vi "Init_graphe.vi"() -> ()   [LabVIEW 2015]
uses:
  <vilib>/Utility/miscctls.llb/LVRowAndColumnTypeDef.ctl
  <vilib>/Utility/file.llb/Read From Spreadsheet File (string).vi
panel:
  in  "Horodatage":timestamp
  in  "Bouton Aide":bool
  in  "Quit":bool
  out "horodatage_ok":timestamp
  in  "Fichier données":path
  out "Colonne données brutes":string="0"
  out "Ligne données brutes":string="0"
  out "Noms variables":string[](array[string])
  out "Séparateur fichier brute":string
  in  "Valider":bool
  in  "Nouveau format date":bool
  in  "Format d'horodatage":string(combo)="\"%Y-%m-%d %H:%M:%S\""
  in  "Convertir Horodatage":bool
  out "Nb lignes":i32
  in  "Séparateur":u16(ring)=1 items=["", ",", ";", ".", "Tab", "Espace", ":"]
  out "Horodatage_1":timestamp[](array[timestamp]) format="%<%X\n%x>T"
  out "Table":string[][](table)
  out "Donnees":dbl[][](array[numeric])
  in  "Bouton vide 2":bool
  # "Facultatif : \nSélectionner la dernière cellule des noms de variables  en appuyant sur la touche CTRL"
  # "Sélectionner la 1ère cellule\ndes noms de variables"
  # "Sélectionner la 1ère cellule\nd'horodatage"
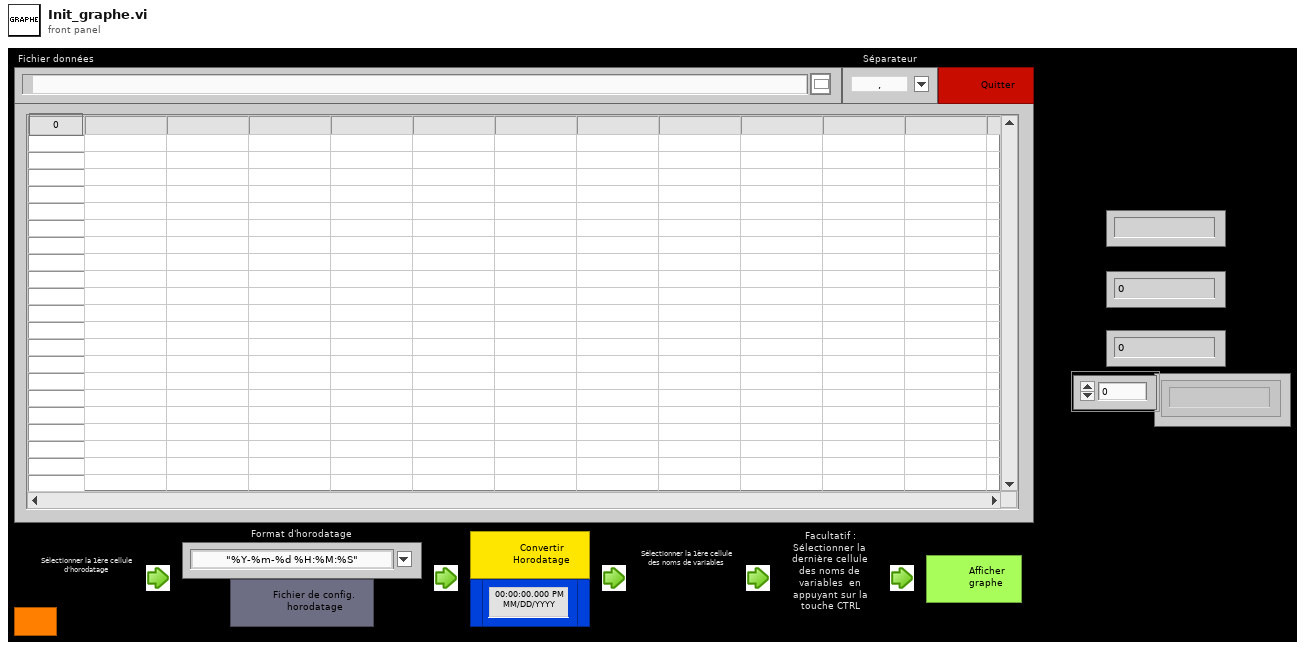
[diagram p1: front panel]
types:
  T1 = typedef "LVRowAndColumnTypeDef.ctl" = cluster{"Row":i32, "Column":i32}
  T2 = typedef "excel Object Reference.ctl" = refnum<k1>
  T3 = enum16{"Left Button", "Center Button", "Right Button", "Window Close"}
  T4 = cluster{"Shift":bool, "Ctrl":bool, "Alt":bool, "Cmd":bool, "Opt":bool}
  T5 = cluster{"Horodatage":timestamp[], "Donnees":dbl[]}[]
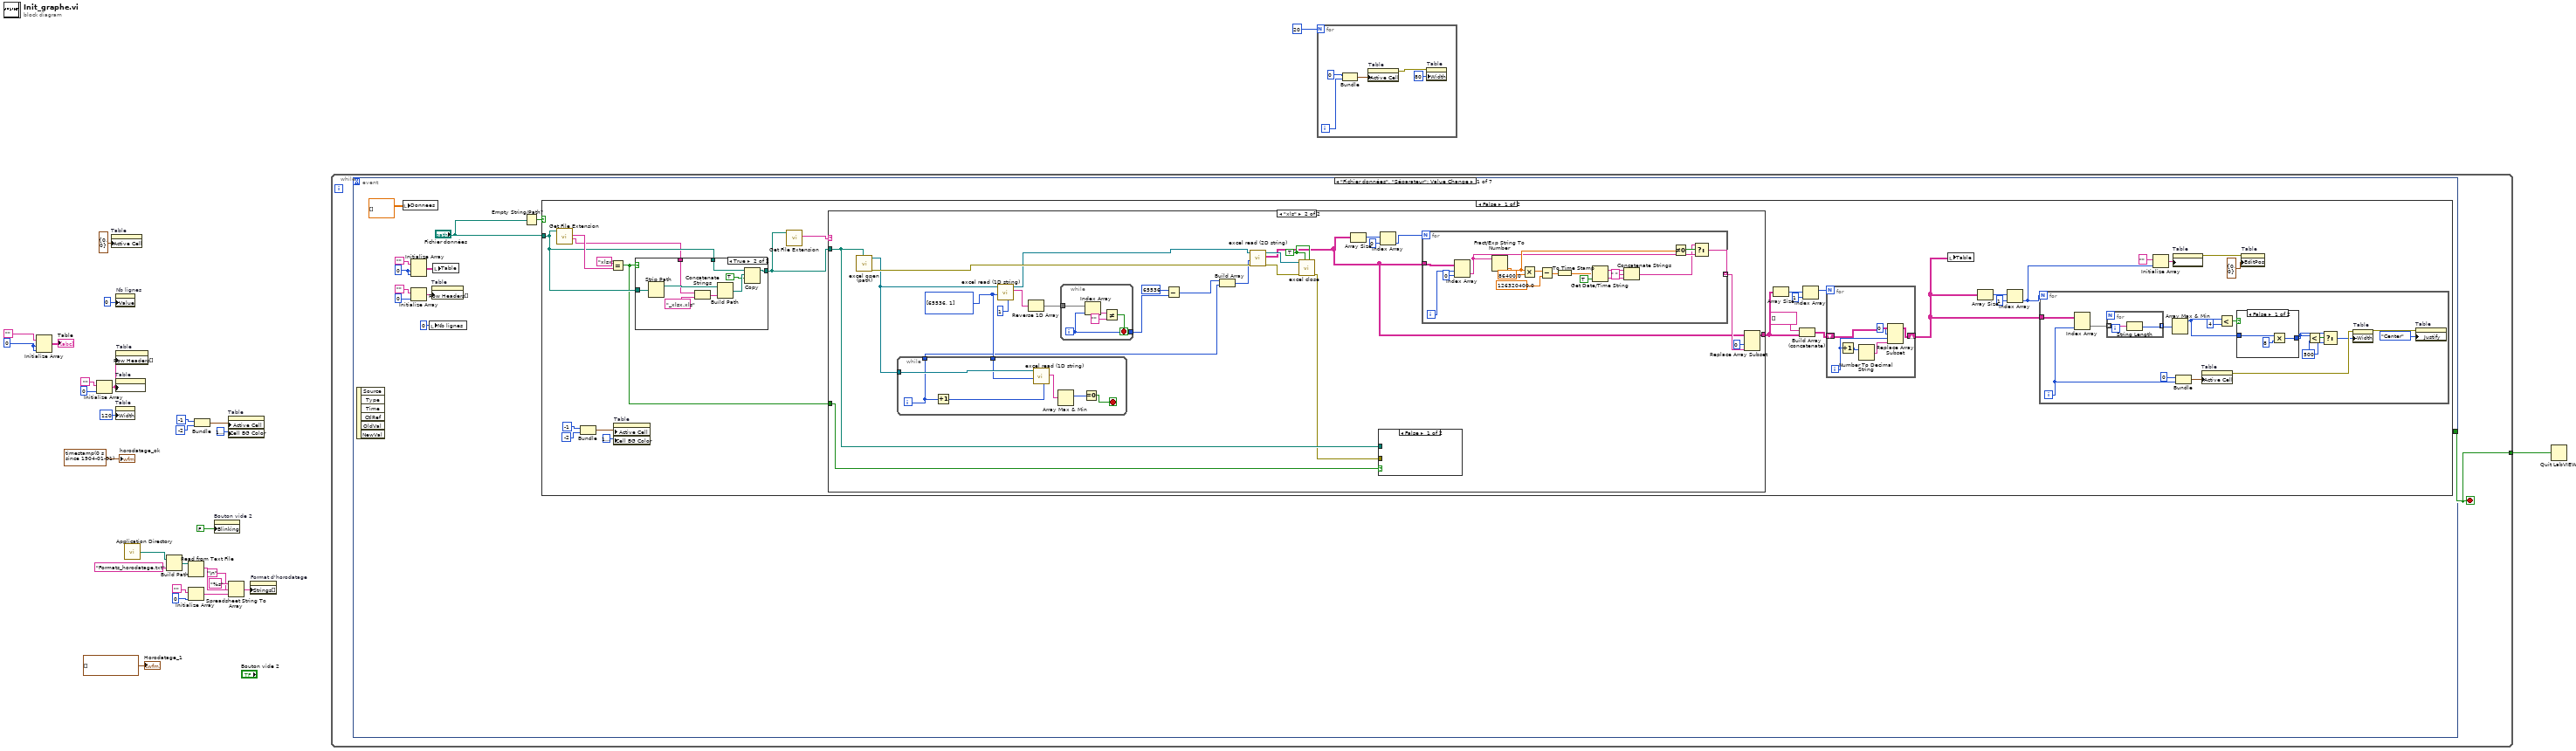
[diagram p0: block diagram]
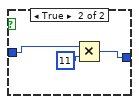
[diagram p3: hidden frame]
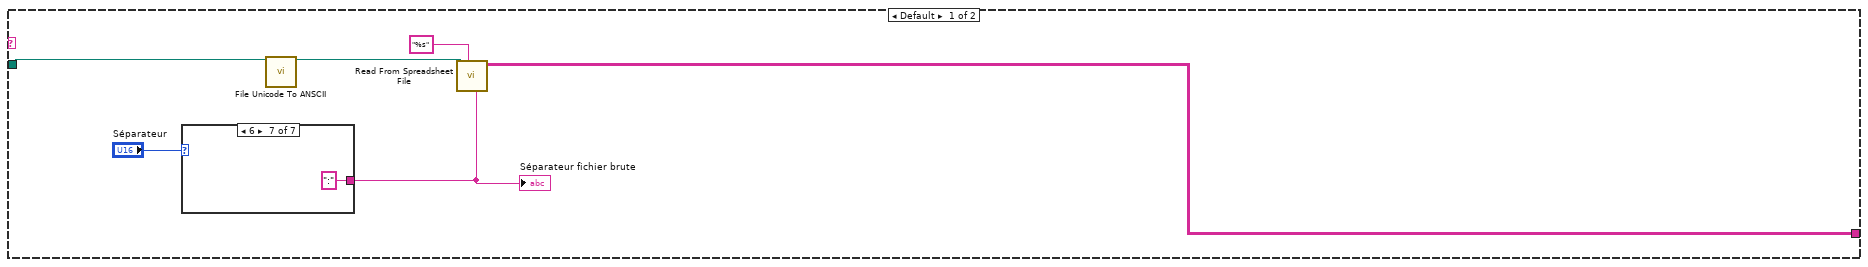
[diagram p4: hidden frame]
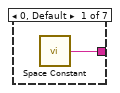
[diagram p5: hidden frame]
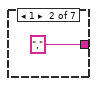
[diagram p6: hidden frame]
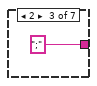
[diagram p7: hidden frame]
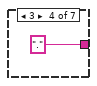
[diagram p8: hidden frame]
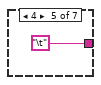
[diagram p9: hidden frame]
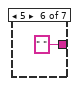
[diagram p10: hidden frame]
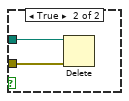
[diagram p11: hidden frame]
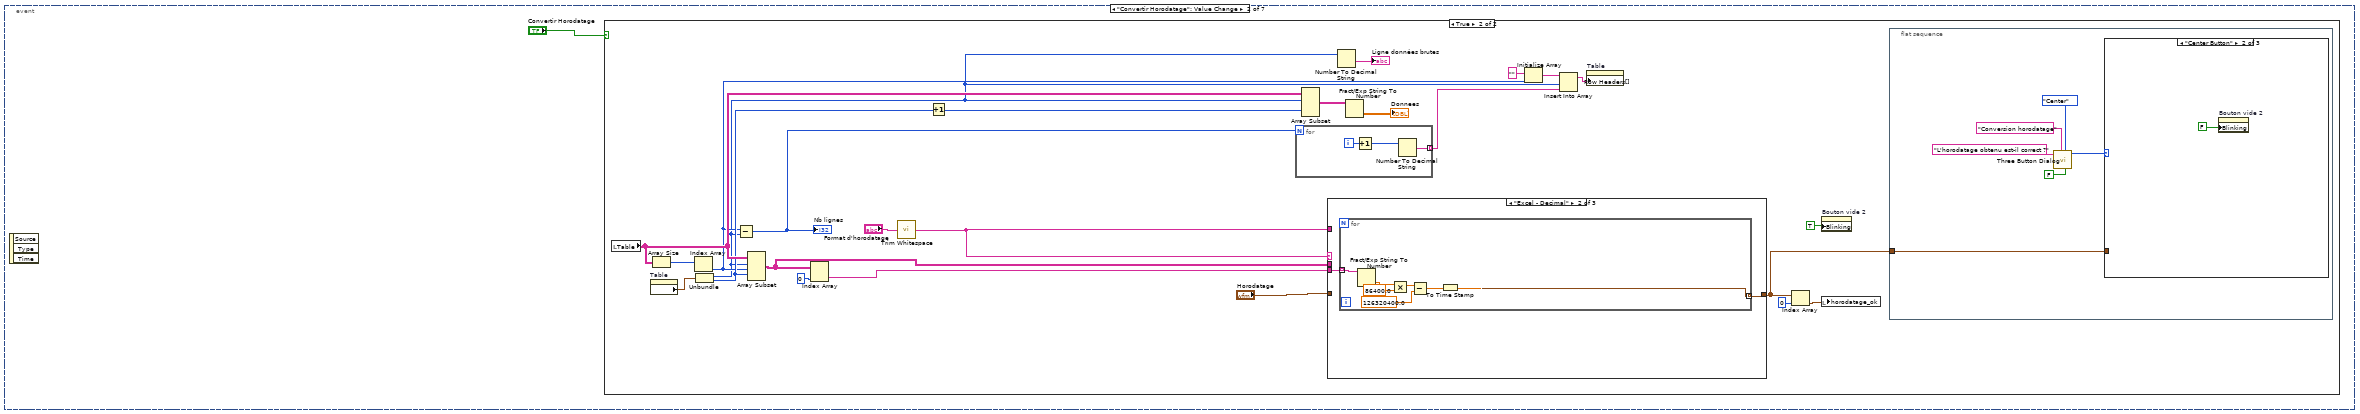
[diagram p13: hidden frame]
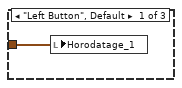
[diagram p15: hidden frame]
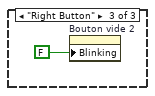
[diagram p16: hidden frame]
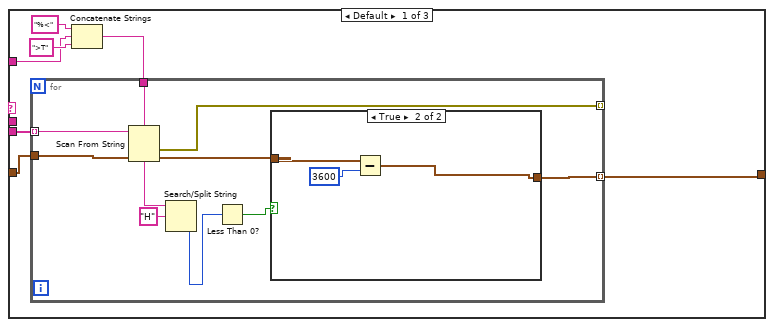
[diagram p17: hidden frame]
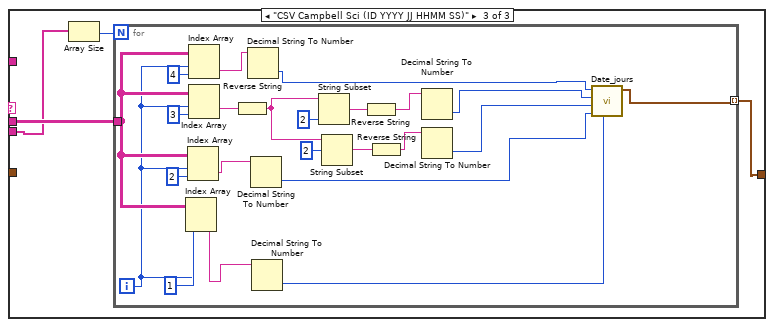
[diagram p19: hidden frame]
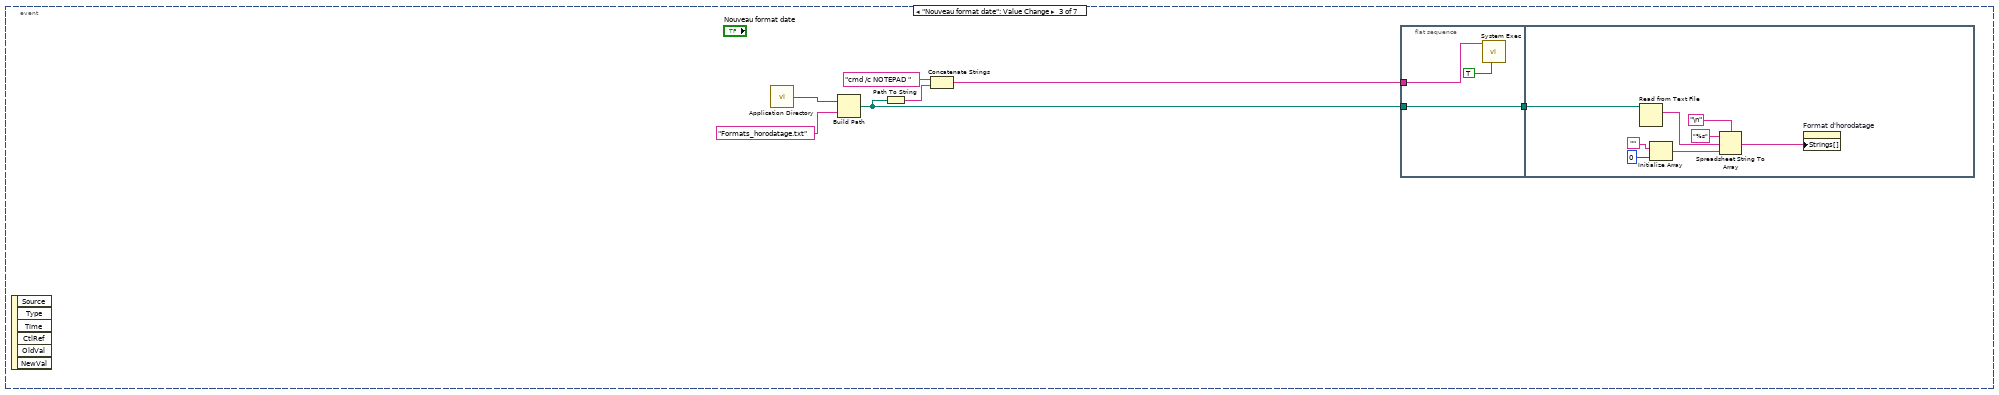
[diagram p20: hidden frame]
diagram:
  w10 = 0 ("taille de la dimension")
  n1 = Initialize Array("", w10, w10) -> (→"Table":string[][])
  n2 = Initialize Array("", 0 ("taille de la dimension")) -> (w17:string[])
  n3 = property on="Table" class="Tbl (strict)"("Active Cell"=T1 {"Row"=0, "Column"=0} ("Cellule active:Cellule active")) -> ()  [unwired: 2 in, 2 out]
  n4 = property on="Table" class="Tbl (strict)"("Column Headers[]"=w17) -> ()  [unwired: 2 in, 2 out]
  n5 = property on="Table" class="Tbl (strict)"("Width"=u32 120 ("Cellule active:Taille de la cellule:Largeur")) -> ()  [unwired: 2 in, 2 out]
  n6 = property on="Nb lignes" class="DigNum (strict)"("Value"=0 ("Nb lignes")) -> ()  [unwired: 2 in, 2 out]
  n7 = property on="Table" class="Tbl (strict)"("Row Headers[]"=w17) -> ()  [unwired: 2 in, 2 out]
  n8 = call <vilib>:"Application Directory.vi"() -> ("Application Directory"=w13:path)
  n9 = Build Path(base path=w13, name or relative path="Formats_horodatage.txt" ("nom ou chemin relatif")) -> (appended path=w21:path)
  n10 = Read from Text File(file (use dialog)=w21) -> (text=w26:string)  [unwired: 3 in, 3 out]
  n11 = Initialize Array("", 0 ("taille de la dimension")) -> (w22:string[])
  n12 = Bundle(-1, -2) -> (w2:cluster{i32, i32})  [unwired: 1 in]
  n13 = property on="Bouton vide 2" class="Bool"("Blinking"=FALSE ("Clignotant")) -> ()  [unwired: 2 in, 2 out]
  n14 = property on="Table" class="Tbl (strict)"("Active Cell"=w2, "Cell BG Color"=u32 16777225) -> ()  [unwired: 2 in, 2 out]
  n15 = Spreadsheet String To Array(delimiter (Tab)="\n", format string="%s" ("chaîne de format"), spreadsheet string=w26, array type (2D Dbl)=w22) -> (array=w18:string[])
  n16 = property on="Format d'horodatage" class="CmbBox"("Strings[]"=w18) -> ()  [unwired: 2 in, 2 out]
  n17 = while {
    tunnel: [w29] -> w7
    stop <- w29 stop-if-true
    n18 = event shown="[0] \"Fichier données\", \"Séparateur\": Value Change" {
      selector: _ -> [_ _ _ _ _ _ _]
      dyn-events: _ -> [_ _ _ _ _ _ _]
      timeout: _ -> [_ _ _ _ _ _ _]
      tunnel: [_ _ _ _ _ w388 _] -> w29
      event "Fichier données", "Séparateur": Value Change {
        w39 = 0 ("taille de la dimension")
        n19 = event-data() -> ()  [unwired: 1 in, 6 out]
        n20 = local write "Donnees"(dbl[][] [] ("Donnees")) -> ()
        n21 = Initialize Array("", w39, w39) -> (w37:string[][])
        n22 = Initialize Array("", 0 ("taille de la dimension")) -> (w34:string[])
        n23 = local write "Nb lignes"(0 ("Nb lignes")) -> ()
        n24 = property on="Table" class="Tbl (strict)"("Row Headers[]"=w34) -> ()  [unwired: 2 in, 2 out]
        n25 = local write "Table"(w37) -> ()
        n26 = Empty String/Path?(string/path="Fichier données") -> (empty?=w31:bool)
        n27 = case shown="False" w31 {
          tunnel: "Fichier données" -> [w44 _]
          frame False {
            n28 = call <vilib>:"Get File Extension.vi"("file"=w44) -> ("filename without extension"=w43:string, "lowercase file extension"=w46:string)  [unwired: 6 in, 3 out]
            n29 = Bundle(-1, -2) -> (w57:cluster{i32, i32})  [unwired: 1 in]
            n30 = Equal?(x="xlsx", y=w46) -> (x = y?=w40:bool)
            n31 = property on="Table" class="Tbl (strict)"("Active Cell"=w57, "Cell BG Color"=u32 16777225) -> ()  [unwired: 2 in, 2 out]
            n32 = case shown="True" w40 {
              tunnel: w44 -> [w65 w74]
              tunnel: [w65 w73] -> w42
              tunnel: w44 -> [_ w71]
              tunnel: w43 -> [_ w68]
              frame False {
              }
              frame True {
                n33 = Strip Path(path=w71) -> (stripped path=w72:path)  [unwired: 1 out]
                n34 = Concatenate Strings(w68, "_xlsx.xls" ("chaîne")) -> (w69:string)
                n35 = Build Path(base path=w72, name or relative path=w69) -> (appended path=w70:path)
                n36 = Copy(9:TRUE ("écraser (F)"), 10:w70, 11:w74) -> (3:w73:path)  [unwired: 2 in, 2 out]
              }
            }
            n37 = call <vilib>:"Get File Extension.vi"("file"=w42) -> ("lowercase file extension"=w41:string)  [unwired: 6 in, 4 out]
            n38 = case shown="\"xls\"" w41 {
              tunnel: w42 -> [w106 w127]
              tunnel: [w108 w128] -> w50
              tunnel: w40 -> [_ w125]
              frame Default {
                n39 = case shown="6" "Séparateur" {
                  tunnel: [w111 "," ";" "." "\t" " " ("String") ":" ("String")] -> w107
                  frame 0, Default {
                    n40 = call <vilib>:"Space Constant.vi"() -> ("String"=w111:string)
                  }
                  frame 1 {
                  }
                  frame 2 {
                  }
                  frame 3 {
                  }
                  frame 4 {
                  }
                  frame 5 {
                  }
                  frame 6 {
                  }
                }
                "Séparateur fichier brute" <- w107
                n41 = call "File Unicode To ANSCII.vi"("file in"=w106) -> ("file out"=w105:path)  [unwired: 18 in]
                n42 = call-poly <vilib>:"Read From Spreadsheet File.vi"("delimiter (\\t)"=w107, "format (%s)"="%s", "file path (dialog if empty)"=w105) -> ("all rows"=w108:string[][])  [unwired: 4 in, 4 out]
              }
              frame "xls" {
                w122 = i32[] [65536, 1] ("array size\n  - #rows\n  - #columns")
                w139 = TRUE ("Override closing behavior")
                n43 = call "excel open (path).vi"("workbook path"=w127) -> ("error out"=w140:errorcluster, "reference"=w124:T2)  [unwired: 9 in]
                n44 = while {
                  tunnel: w124 -> [w148]
                  tunnel: w122 -> [w146]
                  tunnel: [w143] -> w121
                  i -> [w143]
                  stop <- w149 stop-if-true
                  n45 = Increment(x=w143) -> (x+1=w147:i32)
                  n46 = call "excel read (1D string).vi"("Column"=w147, "array size\n  - #rows\n  - #columns"=w146, "reference"=w148) -> ("1D String Array"=w145:string[])  [unwired: 6 in, 2 out]
                  n47 = Array Max & Min(array=w145) -> (max index (indices)=w144:i32)  [unwired: 3 out]
                  n48 = Equal To 0?(x=w144) -> (x = 0?=w149:bool)
                }
                n49 = call "excel read (1D string).vi"("Column"=u32 1, "array size\n  - #rows\n  - #columns"=w122, "reference"=w124) -> ("1D String Array"=w138:string[], "duplicate reference"=w118:T2)  [unwired: 6 in, 1 out]
                n50 = Reverse 1D Array(array=w138) -> (reversed array=w137:string[])
                n51 = while {
                  tunnel: w137 -> [w173]
                  tunnel: [w169] -> w136
                  i -> [w169]
                  stop <- w170 stop-if-true
                  n52 = Index Array(array=w173, index=w169) -> (element=w172:string)
                  n53 = Not Equal?(x=w172, y="") -> (x != y?=w170:bool)
                }
                n54 = Subtract(x=65536, y=w136) -> (x-y=w120:i32)
                n55 = Build Array(w120, w121) -> (w123:i32[])
                n56 = call "excel read (2D string).vi"("error in (no error)"=w140, "array size\n  - #rows\n  - #columns"=w123, "reference"=w118) -> ("error out"=w141:errorcluster, "2D String Array"=w129:string[][], "duplicate reference"=w142:T2)  [unwired: 6 in]
                n57 = call "excel close.vi"("Close"=w139, "Override closing behavior"=w139, "error in (no error)"=w141, "reference"=w142) -> ("error out"=w126:errorcluster)  [unwired: 7 in]
                n58 = Array Size(array=w129) -> (size(s)=w131:i32[])
                n59 = case shown="False" w125 {
                  tunnel: w127 -> [_ w151]
                  tunnel: w126 -> [_ w150]
                  frame False {
                  }
                  frame True {
                    n60 = Delete(path (use dialog)=w151, error in=w150) -> ()  [unwired: 3 in, 3 out]
                  }
                }
                n61 = Index Array(array=w131, index=0 ("indice")) -> (element=w132:i32)
                n62 = for {
                  N: w132 -> [_]
                  tunnel: w129 -> [w168]
                  tunnel: [w153] -> w134 mode=indexing
                  i -> [w167]
                  n63 = Index Array(array=w168, index (row)=w167, index (col)=0 ("indice désactivé (col)")) -> (element=w154:string)
                  n64 = Fract/Exp String To Number(string=w154) -> (number=w155:dbl)  [unwired: 3 in, 1 out]
                  n65 = Multiply(x=w155, y=86400.0) -> (x*y=w164:dbl)
                  n66 = Subtract(x=w164, y=126320400.0) -> (x-y=w162:dbl)
                  n67 = To Time Stamp(1:w162) -> (0:w161:timestamp)
                  n68 = Get Date/Time String(seconds (now)=w161, want seconds? (F)=TRUE ("secondes ? (F)")) -> (date string=w159:string, time string=w157:string)  [unwired: 1 in]
                  n69 = Concatenate Strings(w159, " " ("chaîne"), w157) -> (w152:string)
                  n70 = Not Equal To 0?(x=w155) -> (x != 0?=w156:bool)
                  n71 = Select(t=w152, s=w156, f=w154) -> (s? t:f=w153:string)
                }
                n72 = Replace Array Subset(array=w129, new element=w134, index (col)=0 ("indice désactivé (col)")) -> (w128:string[][])  [unwired: 1 in]
              }
            }
            n73 = Array Size(array=w50) -> (size(s)=w52:i32[])
            n74 = Build Array (concatenate)(string[] [] ("élément"), w50) -> (w48:string[][])
            n75 = Index Array(array=w52, index=1 ("indice")) -> (element=w51:i32)
            n76 = for {
              N: w51 -> [_]
              shift-right: [w80] -> w54
              shift-left: w48 -> [w79]
              i -> [w76]
              n77 = Increment(x=w76) -> (x+1=w78:i32)
              n78 = Number To Decimal String(number=w78) -> (decimal integer string=w75:string)  [unwired: 1 in]
              n79 = Replace Array Subset(array=w79, new element=w75, index (row)=0 ("indice désactivé (ligne)"), index (col)=w76) -> (w80:string[][])
            }
            n80 = local write "Table"(w54) -> ()
            n81 = Array Size(array=w54) -> (size(s)=w60:i32[])
            n82 = Index Array(array=w60, index=1 ("indice")) -> (element=w47:i32)
            n83 = for {
              N: w47 -> [_]
              tunnel: w54 -> [w96]
              i -> [w91]
              w82 = 500 ("cas faux")
              n84 = Index Array(array=w96, index (col)=w91) -> (element=w95:string[])  [unwired: 1 in]
              n85 = for {
                tunnel: w95 -> [w104] mode=indexing
                tunnel: [w103] -> w94 mode=indexing
                n86 = String Length(string=w104) -> (length=w103:i32)
              }
              n87 = Array Max & Min(array=w94) -> (max value=w86:i32)  [unwired: 3 out]
              n88 = Bundle(0, w91) -> (w93:cluster{i32, i32})  [unwired: 1 in]
              n89 = property on="Table" class="Tbl (strict)"("Active Cell"=w93) -> (error out=w92:errorcluster)  [unwired: 2 in, 1 out]
              n90 = Less?(x=w86, y=4) -> (x < y?=w87:bool)
              n91 = case shown="False" w87 {
                tunnel: [w99 w100] -> w81
                tunnel: w86 -> [w97 w101]
                frame False {
                  n92 = Multiply(x=w97, y=8) -> (x*y=w99:i32)
                }
                frame True {
                  n93 = Multiply(x=w101, y=11) -> (x*y=w100:i32)
                }
              }
              n94 = Less?(x=w81, y=w82) -> (x < y?=w83:bool)
              n95 = Select(t=w81, s=w83, f=w82) -> (s? t:f=w84:i32)
              n96 = property on="Table" class="Tbl (strict)"(error in=w92, "Width"=w84) -> (error out=w89:errorcluster)  [unwired: 1 in, 1 out]
              n97 = property on="Table" class="Tbl (strict)"(error in=w89, "Justify"=enum16{"Left", "Center", "Right"}."Center" ("Cellule active:Justification de la cellule")) -> ()  [unwired: 1 in, 2 out]
            }
            n98 = Initialize Array("", w47) -> (w63:string[])
            n99 = property on="Table" class="Tbl (strict)"("Column Headers[]"=w63) -> (error out=w61:errorcluster)  [unwired: 2 in, 1 out]
            n100 = property on="Table" class="Tbl (strict)"(error in=w61, "EditPos"=T1 {"Row"=0, "Column"=0} ("Cellule active:Cellule active")) -> ()  [unwired: 1 in, 2 out]
          }
          frame True {
          }
        }
      }
      event "Convertir Horodatage": Value Change {
        n101 = event-data() -> ()  [unwired: 1 in, 3 out]
        n102 = case shown="True" "Convertir Horodatage" {
          frame False {
          }
          frame True {
            n103 = local read "Table"() -> (w194:string[][])
            n104 = property on="Table" class="Tbl (strict)"() -> ("Selection Start"=w197:T1)  [unwired: 2 in, 2 out]
            n105 = Array Size(array=w194) -> (size(s)=w195:i32[])
            n106 = Index Array(array=w195) -> (element=w189:i32)  [unwired: 1 in]
            n107 = Unbundle(w197) -> ("Row"=w185:i32, "Column"=w190:i32)
            n108 = Subtract(x=w189, y=w185) -> (x-y=w180:i32)
            "Nb lignes" <- w180
            n109 = Array Subset(array=w194, index (row)=w185, length (row)=w189, index (col)=w190) -> (w182:string[][])  [unwired: 1 in]
            n110 = Index Array(array=w182, index (col)=0 ("indice (ligne)")) -> (element=w187:string[])  [unwired: 1 in]
            n111 = call <vilib>:"Trim Whitespace.vi"("string"="Format d'horodatage") -> ("trimmed string"=w176:string)  [unwired: 1 in]
            n112 = Increment(x=w190) -> (x+1=w196:i32)
            n113 = for {
              N: w180 -> [_]
              tunnel: [w266] -> w191 mode=indexing
              i -> [w267]
              n114 = Increment(x=w267) -> (x+1=w265:i32)
              n115 = Number To Decimal String(number=w265) -> (decimal integer string=w266:string)  [unwired: 1 in]
            }
            n116 = Array Subset(array=w194, index (row)=w185, index (col)=w196) -> (w198:string[][])  [unwired: 2 in]
            n117 = case shown="\"Excel - Decimal\"" w176 {
              tunnel: "Horodatage" -> [w215 _ _]
              tunnel: w187 -> [w212 w230 w238]
              tunnel: [w211 w229 w240] -> w179
              tunnel: w176 -> [w209 _ _]
              tunnel: w182 -> [_ _ w241]
              frame Default {
                n118 = Concatenate Strings("%<", w209, ">T") -> (w210:string)
                n119 = for {
                  tunnel: [w219] -> w211 mode=indexing
                  tunnel: w215 -> [w224]
                  tunnel: w210 -> [w222]
                  tunnel: w212 -> [w223] mode=indexing
                  tunnel: [w216] -> _ mode=indexing
                  n120 = Scan From String(format string=w222, input string=w223, default 1=w224) -> (error out=w216:errorcluster, output 1=w220:timestamp)  [unwired: 2 in, 2 out]
                  n121 = Search/Split String(string=w222, search string/char (-)="H" ("chaîne/car. recherché (-)")) -> (offset of match=w218:i32)  [unwired: 1 in, 2 out]
                  n122 = Less Than 0?(x=w218) -> (x < 0?=w217:bool)
                  n123 = case shown="True" w217 {
                    tunnel: w220 -> [w225 w228]
                    tunnel: [w225 w226] -> w219
                    frame False {
                    }
                    frame True {
                      n124 = Subtract(x=w228, y=3600) -> (x-y=w226:timestamp)
                    }
                  }
                }
              }
              frame "Excel - Decimal" {
                n125 = for {
                  tunnel: [w231] -> w229 mode=indexing
                  tunnel: w230 -> [w237] mode=indexing
                  n126 = Fract/Exp String To Number(string=w237) -> (number=w236:dbl)  [unwired: 3 in, 1 out]
                  n127 = Multiply(x=w236, y=86400.0) -> (x*y=w234:dbl)
                  n128 = Subtract(x=w234, y=126320400.0) -> (x-y=w232:dbl)
                  n129 = To Time Stamp(1:w232) -> (0:w231:timestamp)
                }
              }
              frame "CSV Campbell Sci (ID YYYY JJ HHMM SS)" {
                n130 = Array Size(array=w238) -> (size(s)=w239:i32)
                n131 = for {
                  N: w239 -> [_]
                  tunnel: w241 -> [w251]
                  tunnel: [w242] -> w240 mode=indexing
                  i -> [w250]
                  n132 = Index Array(array=w251, index (row)=w250, index (col)=1 ("indice désactivé (col)")) -> (element=w248:string)
                  n133 = Index Array(array=w251, index (row)=w250, index (col)=2 ("indice désactivé (col)")) -> (element=w249:string)
                  n134 = Index Array(array=w251, index (row)=w250, index (col)=4 ("indice désactivé (col)")) -> (element=w263:string)
                  n135 = Index Array(array=w251, index (row)=w250, index (col)=3 ("indice désactivé (col)")) -> (element=w261:string)
                  n136 = Reverse String(1:w261) -> (0:w257:string)
                  n137 = Decimal String To Number(string=w263) -> (number=w247:i32)  [unwired: 2 in, 1 out]
                  n138 = Decimal String To Number(string=w249) -> (number=w244:i32)  [unwired: 2 in, 1 out]
                  n139 = Decimal String To Number(string=w248) -> (number=w243:i32)  [unwired: 2 in, 1 out]
                  n140 = String Subset(string=w257, length (rest)=2 ("longueur (reste)")) -> (substring=w259:string)  [unwired: 1 in]
                  n141 = String Subset(string=w257, offset (0)=2) -> (substring=w255:string)  [unwired: 1 in]
                  n142 = Reverse String(1:w259) -> (0:w258:string)
                  n143 = Reverse String(1:w255) -> (0:w254:string)
                  n144 = Decimal String To Number(string=w258) -> (number=w246:i32)  [unwired: 2 in, 1 out]
                  n145 = Decimal String To Number(string=w254) -> (number=w245:i32)  [unwired: 2 in, 1 out]
                  n146 = call "Date_jours.vi"("year"=w243, "jours n"=w244, "hour"=w245, "minute"=w246, "second"=w247) -> ("horodatage"=w242:timestamp)  [unwired: 6 in]
                }
              }
            }
            n147 = Number To Decimal String(number=w185) -> (decimal integer string=→"Ligne données brutes":string)  [unwired: 1 in]
            n148 = Fract/Exp String To Number(string=w198) -> (number=→"Donnees":dbl[][])  [unwired: 3 in, 1 out]
            n149 = Initialize Array("", w189) -> (w192:string[])
            n150 = Insert Into Array(array=w192, index=w185, new element=w191) -> (w181:string[])
            n151 = property on="Table" class="Tbl (strict)"("Row Headers[]"=w181) -> ()  [unwired: 2 in, 2 out]
            n152 = Index Array(array=w179, index=0 ("indice")) -> (element=w178:timestamp)
            n153 = local write "horodatage_ok"(w178) -> ()
            n154 = property on="Bouton vide 2" class="Bool"("Blinking"=TRUE ("Clignotant")) -> ()  [unwired: 2 in, 2 out]
            n155 = flat-sequence {
              tunnel: w179 -> [w200]
              frame #0 {
                n156 = call <vilib>:"Three Button Dialog.vi"("Allow user to close window? (TRUE)"=FALSE, "Justify Message (Left)"=enum16{"Left", "Center", "Right"}."Center", "Window Title (\"\")"="Conversion horodatage" ("error source (\" \")"), "message"="L'horodatage obtenu est-il correct ?" ("error source (\" \")")) -> ("Which Button?"=w203:T3)  [unwired: 7 in]
                n157 = case shown="\"Center Button\"" w203 {
                  tunnel: w200 -> [w206 _ _]
                  frame "Left Button", Default {
                    n158 = local write "Horodatage_1"(w206) -> ()
                  }
                  frame "Center Button" {
                    n159 = property on="Bouton vide 2" class="Bool"("Blinking"=FALSE ("Clignotant")) -> ()  [unwired: 2 in, 2 out]
                  }
                  frame "Right Button" {
                    n160 = property on="Bouton vide 2" class="Bool"("Blinking"=FALSE ("Clignotant")) -> ()  [unwired: 2 in, 2 out]
                  }
                }
              }
            }
          }
        }
      }
      event "Nouveau format date": Value Change {
        n161 = event-data() -> ()  [unwired: 1 in, 6 out]
        n162 = call <vilib>:"Application Directory.vi"() -> ("Application Directory"=w268:path)
        n163 = Build Path(base path=w268, name or relative path="Formats_horodatage.txt" ("nom ou chemin relatif")) -> (appended path=w270:path)
        n164 = Path To String(path=w270) -> (string=w271:string)
        n165 = Concatenate Strings("cmd /c NOTEPAD " ("command line"), w271) -> (w273:string)
        n166 = flat-sequence {
          tunnel: w273 -> [w277]
          tunnel: w270 -> [w275]
          tunnel: [w275] -> w269
          tunnel: w269 -> [w278]
          frame #0 {
            n167 = call <vilib>:"System Exec.vi"("run minimized? (F)"=TRUE, "command line"=w277) -> ()  [unwired: 6 in, 4 out]
          }
          frame #1 {
            n168 = Read from Text File(file (use dialog)=w278) -> (text=w279:string)  [unwired: 3 in, 3 out]
            n169 = Initialize Array("", 0 ("taille de la dimension")) -> (w283:string[])
            n170 = Spreadsheet String To Array(delimiter (Tab)="\n", format string="%s" ("chaîne de format"), spreadsheet string=w279, array type (2D Dbl)=w283) -> (array=w285:string[])
            n171 = property on="Format d'horodatage" class="CmbBox"("Strings[]"=w285) -> ()  [unwired: 2 in, 2 out]
          }
        }
      }
      event "Table": Mouse Down {
        n172 = event-data() -> ("PlatMods"=w293:T4)  [unwired: 1 in, 7 out]
        n173 = local read "Horodatage_1"() -> (w292:timestamp[])
        n174 = property on="Table" class="Tbl (strict)"() -> ("Selection Start"=w288:T1)  [unwired: 2 in, 2 out]
        n175 = Array Size(array=w292) -> (size(s)=w291:i32)
        n176 = Equal To 0?(x=w291) -> (x = 0?=w289:bool)
        n177 = Unbundle(w288) -> ("Column"=w287:i32)  [unwired: 1 out]
        n178 = Equal To 0?(x=w287) -> (x = 0?=w286:bool)
        n179 = Or(x=w286, y=w289) -> (x .or. y?=w290:bool)
        n180 = case shown="False" w290 {
          tunnel: w293 -> [w300 _]
          frame False {
            n181 = Unbundle(w300) -> ("Ctrl"=w299:bool)  [unwired: 4 out]
            n182 = case shown="True" w299 {
              tunnel: [w324 w343] -> w296
              tunnel: [w322 w343] -> w295
              frame False {
                n183 = local read "Table"() -> (w321:string[][])
                n184 = property on="Table" class="Tbl (strict)"() -> ("Selection Start"=w323:T1)  [unwired: 2 in, 2 out]
                n185 = Array Size(array=w321) -> (size(s)=w334:i32[])
                n186 = Unbundle(w323) -> ("Row"=w325:i32, "Column"=w327:i32)
                n187 = Index Array(array=w334, index=1 ("indice")) -> (element=w328:i32)
                n188 = Subtract(x=w328, y=w327) -> (x-y=w332:i32)
                n189 = Number To Decimal String(number=w327) -> (decimal integer string=→"Colonne données brutes":string)  [unwired: 1 in]
                n190 = Array Subset(array=w321, index (row)=w325, length (row)=1 ("longueur"), index (col)=w327, length (col)=w332) -> (w335:string[][])
                n191 = Index Array(array=w335, index (row)=0 ("indice (ligne)")) -> (element=w324:string[])  [unwired: 1 in]
                n192 = Initialize Array("", w328) -> (w330:string[])
                n193 = Replace Array Subset(array=w330, new element=w324, index=w327) -> (w322:string[])
                n194 = property on="Table" class="Tbl (strict)"("Column Headers[]"=w322) -> ()  [unwired: 2 in, 2 out]
              }
              frame True {
                n195 = Bundle(-1, -2) -> (w340:cluster{i32, i32})  [unwired: 1 in]
                n196 = property on="Table" class="Tbl (strict)"("Active Cell"=w340, "Cell BG Color"=u32 16777225) -> ()  [unwired: 2 in, 2 out]
                n197 = property on="Table" class="Tbl (strict)"() -> ("Column Headers[]"=w342:string[], "Selection Start"=w337:T1)  [unwired: 2 in, 2 out]
                n198 = Unbundle(w337) -> ("Column"=w344:i32)  [unwired: 1 out]
                n199 = Increment(x=w344) -> (x+1=w346:i32)
                n200 = Array Subset(array=w342, index=0 ("indice"), length=w346) -> (w343:string[])
                n201 = property on="Table" class="Tbl (strict)"("Column Headers[]"=w343) -> ()  [unwired: 2 in, 2 out]
              }
            }
            n202 = for {
              tunnel: w296 -> [w309] mode=indexing
              shift-right: [w311] -> w298
              shift-left: string[] [] -> [w312]
              n203 = Search and Replace String(replace all?=TRUE ("tout remplacer ? (F)"), input string=w309, search string="\"" ("chaîne recherchée"), replace string="" ("chaîne de remplacement (\"\")")) -> (result string=w310:string)  [unwired: 4 in, 3 out]
              n204 = Empty String/Path?(string/path=w310) -> (empty?=w313:bool)
              n205 = case shown="True" w313 {
                tunnel: w312 -> [w319 w320]
                tunnel: [w317 w320] -> w311
                tunnel: w310 -> [w318 _]
                frame False {
                  n206 = Build Array (concatenate)(w319, w318) -> (w317:string[])
                }
                frame True {
                }
              }
            }
            "Noms variables" <- w298
            n207 = for {
              tunnel: w295 -> [w308] mode=indexing
              i -> [w306]
              n208 = Empty String/Path?(string/path=w308) -> (empty?=w304:bool)
              n209 = Bundle(-1, w306) -> (w305:cluster{i32, i32})  [unwired: 1 in]
              n210 = Select(t=u32 16777225, s=w304, f=u32 10473471) -> (s? t:f=w301:u32)
              n211 = property on="Table" class="Tbl (strict)"("Active Cell"=w305, "Cell BG Color"=w301) -> ()  [unwired: 2 in, 2 out]
            }
          }
          frame True {
          }
        }
        n212 = property on="Table" class="Tbl (strict)"("Selection Size"=T1 {"Row"=1, "Column"=1} ("Taille de sélection")) -> ()  [unwired: 2 in, 2 out]
      }
      event "Valider": Value Change {
        n213 = event-data() -> ()  [unwired: 1 in, 6 out]
        n214 = property on="Table" class="Tbl (strict)"() -> ("Column Headers[]"=w352:string[])  [unwired: 2 in, 2 out]
        n215 = local read "Horodatage_1"() -> (w357:timestamp[])
        n216 = Sort 1D Array(array=w352) -> (sorted array=w351:string[])
        n217 = Array Size(array=w357) -> (size(s)=w356:i32)
        n218 = Reverse 1D Array(array=w351) -> (reversed array=w347:string[])
        n219 = Not Equal To 0?(x=w356) -> (x != 0?=w353:bool)
        n220 = Index Array(array=w347) -> (element=w350:string)  [unwired: 1 in]
        n221 = property on="Table" class="Tbl (strict)"("Selection Size"=T1 {"Row"=1, "Column"=1} ("Taille de sélection")) -> ()  [unwired: 2 in, 2 out]
        n222 = Empty String/Path?(string/path=w350) -> (empty?=w349:bool)
        n223 = Not(x=w349) -> (.not. x?=w348:bool)
        n224 = And(x=w348, y=w353) -> (x .and. y?=w354:bool)
        n225 = case shown="True" w354 {
          tunnel: "Valider" -> [_ w365]
          tunnel: w357 -> [_ w364]
          frame False {
            w361 = "" ("Left Button Text (\"Yes\")")
            n226 = call <vilib>:"Three Button Dialog.vi"("Justify Message (Left)"=enum16{"Left", "Center", "Right"}."Center", "Window Title (\"\")"="Problème affichage graphe" ("Window Title (\"\")"), "Right Button Text (\"Cancel\")"=w361, "Center Button Text (\"No\")"="Ok" ("Center Button Text (\"No\")"), "Left Button Text (\"Yes\")"=w361, "message"="Veuillez convertir les dates - heures\net sélectionner au moins une variable\npour afficher le graphe") -> ()  [unwired: 5 in, 1 out]
          }
          frame True {
            n227 = case shown="True" w365 {
              tunnel: w364 -> [_ w371]
              frame False {
              }
              frame True {
                n228 = local read "Table"() -> (w381:string[][])
                n229 = property on="Table" class="Tbl (strict)"() -> ("Selection Start"=w367:T1)  [unwired: 2 in, 2 out]
                n230 = Array Size(array=w381) -> (size(s)=w380:i32[])
                n231 = Unbundle(w367) -> ("Row"=w376:i32, "Column"=w375:i32)
                n232 = Index Array(array=w380, index=1 ("indice")) -> (element=w372:i32)
                n233 = Subtract(x=w372, y=w375) -> (x-y=w378:i32)
                n234 = Array Subset(array=w381, index (row)=w376, length (row)=1 ("longueur"), index (col)=w375, length (col)=w378) -> (w383:string[][])
                n235 = Index Array(array=w383, index (row)=0 ("indice (ligne)")) -> (element=w370:string[])  [unwired: 1 in]
                n236 = Initialize Array("", w372) -> (w374:string[])
                n237 = Replace Array Subset(array=w374, new element=w370, index=w375) -> ()  [unwired: 1 out]
                n238 = local read "Donnees"() -> (w382:dbl[][])
                n239 = property on="Table" class="Tbl (strict)"() -> ("Column Headers[]"=w366:string[])  [unwired: 2 in, 2 out]
                n240 = call "MAJ_Graphe.vi"("Horodatage"=w371, "Donnees"=w382, "Entetes colonnes"=w366) -> ("Graphe"=w369:T5, "Paramètres à afficher"=w368:string[])  [unwired: 5 in]
                n241 = flat-sequence {
                  tunnel: w369 -> [w386]
                  tunnel: w368 -> [w385]
                  frame #0 {
                    n242 = call "Graphe_XY.vi"("Graphe"=w386, "Tableau de chaînes"=w385) -> ()  [unwired: 9 in]
                  }
                  frame #1 {
                    n243 = property on="Table" class="Tbl (strict)"("Active Cell"=T1 {"Row"=0, "Column"=0} ("Cellule active:Cellule active")) -> ()  [unwired: 2 in, 2 out]
                  }
                }
              }
            }
          }
        }
      }
      event "Quit": Value Change {
        n244 = event-data() -> ("NewVal"=w388:bool)  [unwired: 1 in, 5 out]
      }
      event "Bouton Aide": Value Change {
        n245 = event-data() -> ()  [unwired: 1 in, 6 out]
        n246 = call <vilib>:"Application Directory.vi"() -> ("Application Directory"=w390:path)
        n247 = Build Path(base path=w390, name or relative path="Logiciel GRAPHE_Instruction.pdf" ("standard input")) -> (appended path=w389:path)
        n248 = call "Open PDF.vi"("Path"=w389) -> ()  [unwired: 5 in, 2 out]
      }
    }
  }
  n249 = for {
    N: 20 -> [_]
    i -> [w394]
    n250 = Bundle(0, w394) -> (w395:cluster{i32, i32})  [unwired: 1 in]
    n251 = property on="Table" class="Tbl (strict)"("Active Cell"=w395) -> (error out=w392:errorcluster)  [unwired: 2 in, 1 out]
    n252 = property on="Table" class="Tbl (strict)"(error in=w392, "Width"=u32 80 ("Cellule active:Taille de la cellule:Largeur")) -> ()  [unwired: 1 in, 2 out]
  }
  n253 = Quit LabVIEW(quit? (T)=w7) -> ()
  "Horodatage_1" <- timestamp[] [] ("Horodatage")
  "horodatage_ok" <- timestamp(0 s since 1904-01-01)
